vi "2DBangBang.vi"(0 "object in":refnum<class "Navigation.lvclass">, 1 "acceleration":dbl=2.5, 2 "Robot":refnum<class "Robot.lvclass">, 3 "Dest_array":T1(array[cluster]), 4 "Game":refnum<class "Game.lvclass">, 5 "error in (no error)":errorcluster) -> (14 "object out":refnum<class "Navigation.lvclass">, 16 "Robot 2":refnum<class "Robot.lvclass">, 19 "error out":errorcluster)   [LabVIEW 2023, in "Navigation.lvclass"]
uses:
  Navigation.lvclass
  Robot_class/Robot.lvclass
  C:/Users/ebert/Desktop/roboime/SSL_AI/Object_class/Object.lvclass
  Game_class/Game.lvclass
  Team_class/KeeperPlay.ctl
  Game_class/Game.lvclass/Game.ctl
  Team_class/Team.lvclass/Team.ctl
  Parameters_class/Parameters.lvclass/Parameters.ctl
  Robot_class/Robot.lvclass/Robot.ctl
  Object_class/Object.lvclass/Object.ctl
  <vilib>/Analysis/coordinate.llb/2D Cartesian Coordinate Rotation (Scalar).vi
  <vilib>/Analysis/baseanly.llb/Unit Vector (DBL).vi
  Game_class/Read KeeperTeam.vi
  Game_class/Read Parameters.lvclass.vi
  Parameters_class/Read Debug.vi
  Team_class/Read KeeperPlay.vi
  Robot_class/Read orientation.vi
  Robot_class/Read dest_vel.vi
  Object_class/Read x.vi
  Object_class/Read y.vi
  Object_class/Read position(x,y).vi
  Robot_class/Write v_tang.vi
  Robot_class/Write v_norm.vi
  Robot_class/Write v_ang.vi
  Ally_class/Ally.lvclass
  C:/Users/ebert/Desktop/roboime/SSL_AI/Team_class/Team.lvclass
  Parameters_class/Parameters.lvclass
  <vilib>/Analysis/NI_AALPro.lvlib
  <vilib>/Analysis/NI_AALBase.lvlib
panel:
  in  "vMax":dbl=4.0 format="%#_13g"
  in  "maxAngle":dbl=5.0 format="%#_13g"
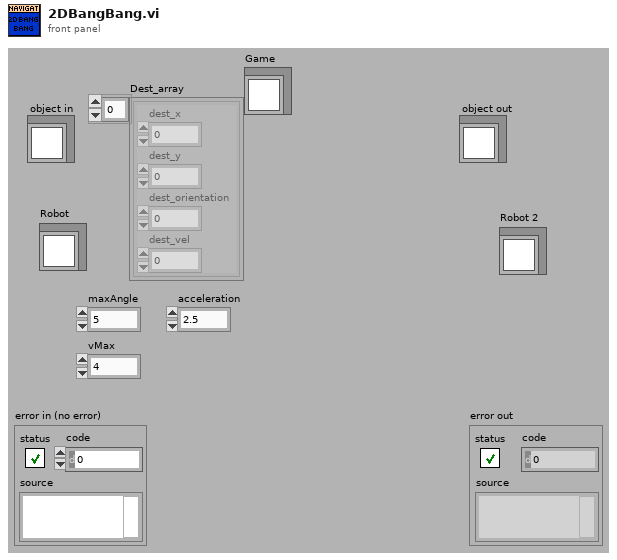
[diagram p1: front panel]
types:
  T1 = cluster{"dest_x":dbl, "dest_y":dbl, "dest_orientation":dbl, "dest_vel":dbl}[]
  T2 = typedef "KeeperPlay.ctl" = enum16{"SimpleBallPlacementAlly", "BallPlacementAlly", "BallPlacementEnemy", "ZigZag", "Goto", "NormalGame", "KeeperPlay", "Halt", "Timeout", "PenaltyEnemy", "TestPlay"}
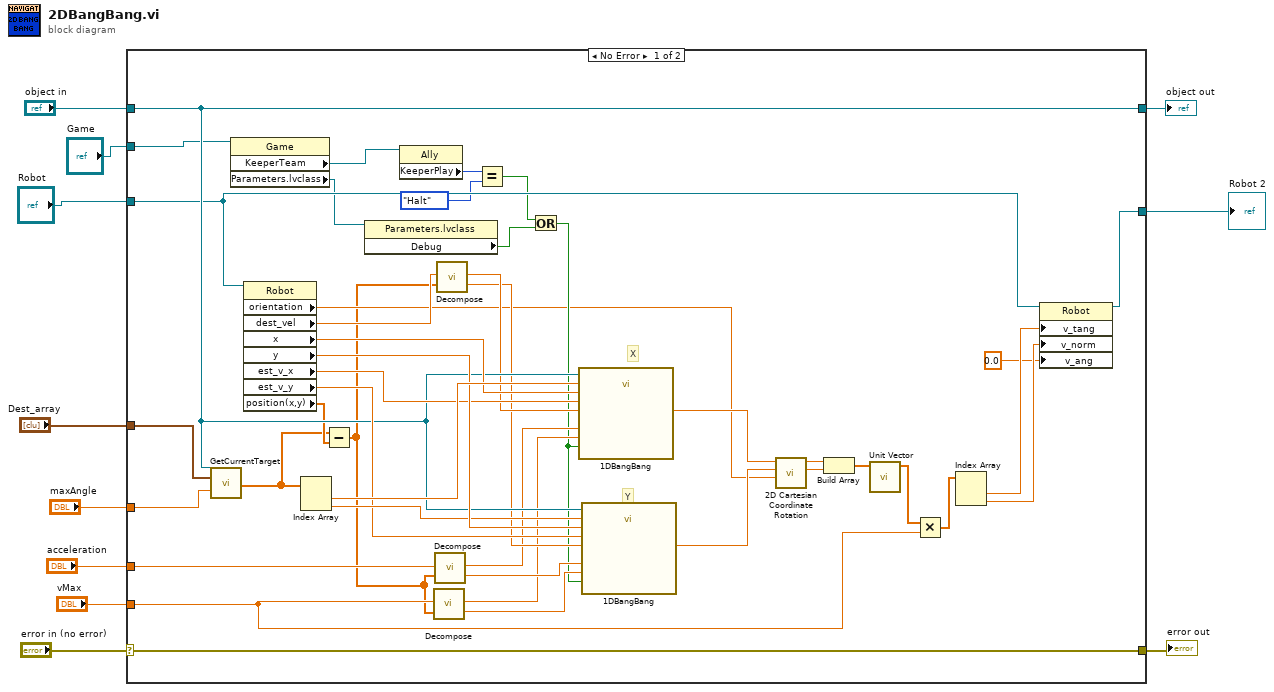
[diagram p0: block diagram]
diagram:
  n1 = case shown="No Error" "error in (no error)" {
    selector: "error in (no error)" -> [w54 w57]
    tunnel: [w54 w57] -> w10
    tunnel: [w45 w56] -> w8
    tunnel: "object in" -> [w45 w56]
    tunnel: "Robot" -> [w26 w55]
    tunnel: "Dest_array" -> [w53 _]
    tunnel: "maxAngle" -> [w52 _]
    tunnel: "acceleration" -> [w40 _]
    tunnel: "vMax" -> [w30 _]
    tunnel: [w25 w55] -> w2
    tunnel: "Game" -> [w22 _]
    frame No Error {
      # "Y"
      # "X"
      n2 = call-dynamic "GetCurrentTarget.vi"("object in"=w45, "Dest_array"=w53, "maxAngle"=w52) -> ("Target"=w39:dbl[])  [unwired: 14 in, 2 out]
      n3 = property class="Game"(reference=w22) -> ("KeeperTeam"=w21:refnum<class "Ally.lvclass">, "Parameters.lvclass"=w17:refnum<class "Parameters.lvclass">)  [unwired: 1 in, 2 out]
      n4 = property class="Robot"(reference=w26) -> ("orientation"=w13:dbl, "dest_vel"=w44:dbl, "x"=w50:dbl, "y"=w49:dbl, "est_v_x"=w47:dbl, "est_v_y"=w46:dbl, "position(x,y)"=w43:dbl[])  [unwired: 1 in, 2 out]
      n5 = Index Array(array=w39) -> (element #1=w51:dbl, element #2=w48:dbl)  [unwired: 2 in]
      n6 = Subtract(x=w39, y=w43) -> (x-y=w12:dbl[])
      n7 = property class="Parameters.lvclass"(reference=w17) -> ("Debug"=w16:bool)  [unwired: 1 in, 2 out]
      n8 = property class="Ally"(reference=w21) -> ("KeeperPlay"=w20:T2)  [unwired: 1 in, 2 out]
      n9 = call "Decompose.vi"("value"=w30, "vector"=w12) -> ("xValue"=w36:dbl, "yValue"=w35:dbl)  [unwired: 14 in, 2 out]
      n10 = call "Decompose.vi"("value"=w40, "vector"=w12) -> ("xValue"=w38:dbl, "yValue"=w37:dbl)  [unwired: 14 in, 2 out]
      n11 = call "Decompose.vi"("value"=w44, "vector"=w12) -> ("xValue"=w42:dbl, "yValue"=w41:dbl)  [unwired: 14 in, 2 out]
      n12 = Equal?(x=w20, y=KeeperPlay."Halt") -> (x = y?=w18:bool)
      n13 = Or(x=w18, y=w16) -> (x .or. y?=w15:bool)
      n14 = call-dynamic "1DBangBang.vi"("object in"=w45, "Target"=w51, "Position"=w50, "curVel"=w47, "destVel"=w42, "Stop"=w15, "acceleration"=w38, "v_max"=w36) -> ("outputVel"=w34:dbl)  [unwired: 9 in, 2 out]
      n15 = call-dynamic "1DBangBang.vi"("object in"=w45, "Target"=w48, "Position"=w49, "curVel"=w46, "destVel"=w41, "Stop"=w15, "acceleration"=w37, "v_max"=w35) -> ("outputVel"=w33:dbl)  [unwired: 9 in, 2 out]
      n16 = call-poly <vilib>:"2D Cartesian Coordinate Rotation.vi"("theta"=w13, "y"=w33, "x"=w34) -> ("y out"=w31:dbl, "x out"=w32:dbl)  [unwired: 6 in, 1 out]
      n17 = Build Array(w32, w31) -> (w28:dbl[])
      n18 = call-poly <vilib>:"Unit Vector.vi"("Input Vector"=w28) -> ("Unit Vector"=w27:dbl[])  [unwired: 8 in, 2 out]
      n19 = Multiply(x=w27, y=w30) -> (x*y=w29:dbl[])
      n20 = Index Array(array=w29) -> (element #1=w24:dbl, element #2=w23:dbl)  [unwired: 2 in]
      n21 = property class="Robot"(reference=w26, "v_tang"=w24, "v_norm"=w23, "v_ang"=0.0) -> (reference out=w25:refnum<class "Robot.lvclass">)  [unwired: 1 in, 1 out]
    }
    frame Error {
    }
  }
  "error out" <- w10
  "object out" <- w8
  "Robot 2" <- w2
